vi "test--get the control data.vi"   [LabVIEW 2021]
doc: "test VI to load the control data.\n\n<b>Code Developed By:</b>\nTechnology Service Corporation\nwww.tsc.com/atcs\n\nDeveloper:\nDaniel Coons"
panel:
  # "Run ME"
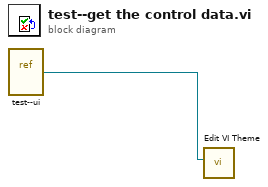
[diagram p0: block diagram]
diagram:
  n1 = vi-ref "test--ui.vi"() -> (w1:refnum<vi>)
  n2 = call "Edit VI Theme.vi"("VI Refnum"=w1) -> ()  [unwired: 11 in]
